vi "GenerateScanPixelMap.vi"(8 "error in":errorcluster, 9 "Mode":enum16{"Raster", "Serpentine"}(ring), 10 "Line Count":i32=6, 11 "Pixel Count":i32=6) -> (0 "error out":errorcluster, 3 "Coordinate Array":i32[][](array[numeric]))   [LabVIEW 2020]
panel:
  out "Pixel Map":cluster{i32[], i32[]}(graph)
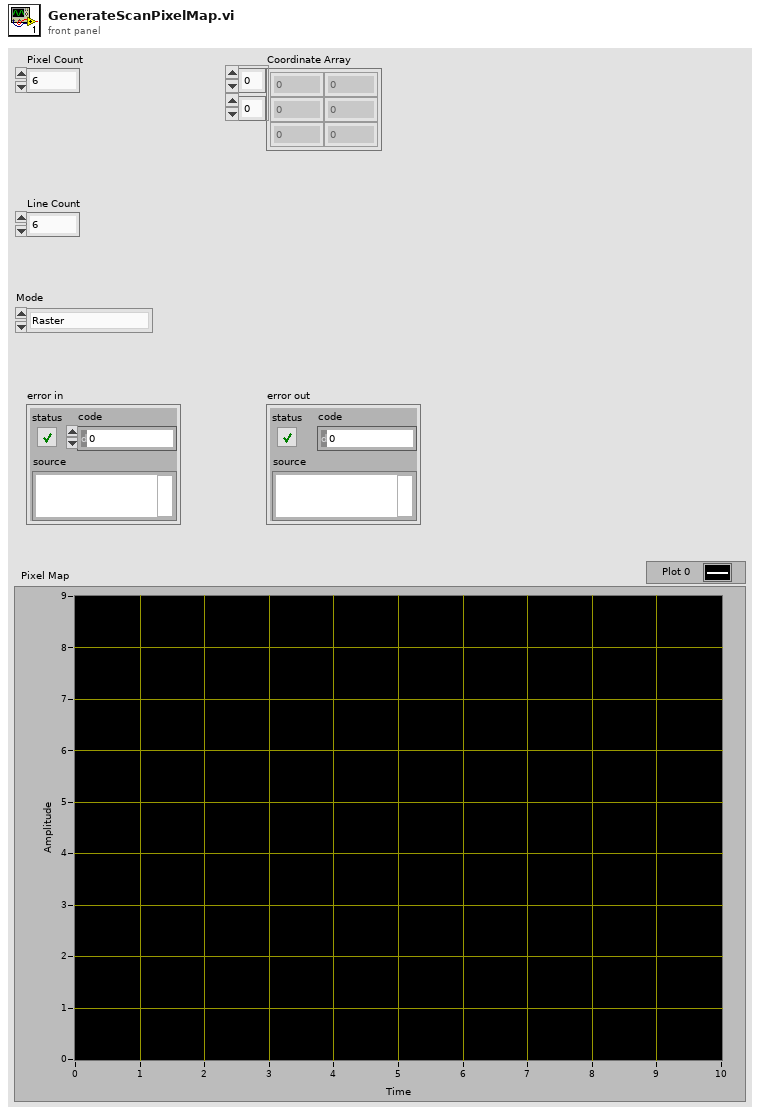
[diagram p1: front panel]
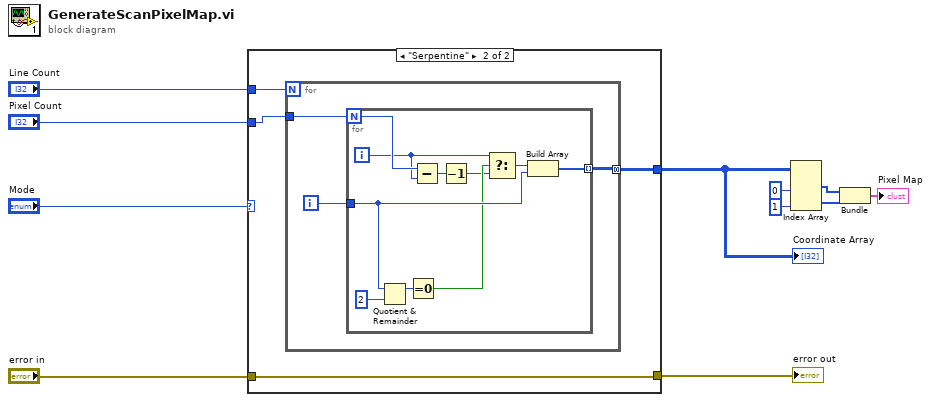
[diagram p0: block diagram]
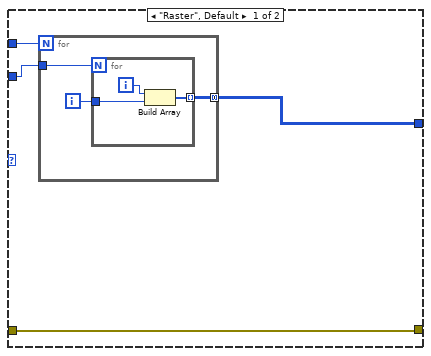
[diagram p2: hidden frame]
diagram:
  n1 = case shown="\"Serpentine\"" "Mode" {
    tunnel: "Line Count" -> [w15 w25]
    tunnel: "Pixel Count" -> [w14 w24]
    tunnel: [w13 w23] -> w5
    tunnel: [w12 w22] -> w1
    tunnel: "error in" -> [w12 w22]
    frame "Raster", Default {
      n2 = for {
        N: w15 -> [_]
        tunnel: w14 -> [w18]
        tunnel: [w16] -> w13 mode=concatenating
        i -> [w17]
        n3 = for {
          N: w18 -> [_]
          tunnel: w17 -> [w19]
          tunnel: [w20] -> w16 mode=indexing
          i -> [w21]
          n4 = Build Array(w21, w19) -> (w20:i32[])
        }
      }
    }
    frame "Serpentine" {
      n5 = for {
        N: w25 -> [_]
        tunnel: w24 -> [w28]
        tunnel: [w26] -> w23 mode=concatenating
        i -> [w27]
        n6 = for {
          N: w28 -> [w31]
          tunnel: w27 -> [w37]
          tunnel: [w38] -> w26 mode=indexing
          i -> [w30]
          n7 = Quotient & Remainder(x=w37, y=2) -> (x-y*floor(x/y)=w35:i32)  [unwired: 1 out]
          n8 = Equal To 0?(x=w35) -> (x = 0?=w34:bool)
          n9 = Subtract(x=w31, y=w30) -> (x-y=w32:i32)
          n10 = Decrement(x=w32) -> (x-1=w29:i32)
          n11 = Select(t=w30, s=w34, f=w29) -> (s? t:f=w33:i32)
          n12 = Build Array(w33, w37) -> (w38:i32[])
        }
      }
    }
  }
  "Coordinate Array" <- w5
  "error out" <- w1
  n13 = Index Array(array=w5, index (col) #1=0 ("disabled index (col)"), index (col) #2=1 ("index (col)")) -> (element #1=w9:i32[], element #2=w8:i32[])  [unwired: 2 in]
  n14 = Bundle(w9, w8) -> (→"Pixel Map":cluster{i32[], i32[]})  [unwired: 1 in]
